vi "start.vi"(5 "FPS":dbl=1000.0, 6 "error in (no error)":errorcluster, 7 "Exposure (ms)":dbl=0.001, 8 "Cam id":u32, 9 "session in":refnum<k35>) -> (0 "error out":errorcluster, 1 "return value":T1={"x"=2592, "y"=1944, "FPS"=30.757874015748033, "Exposure"=0.027793333333333333}, 3 "session out":refnum<k35>)   [LabVIEW 2022 SP3]
panel:
  in  "Image Size template":T1={"x"=2592, "y"=1944, "FPS"=0.0, "Exposure"=0.0}
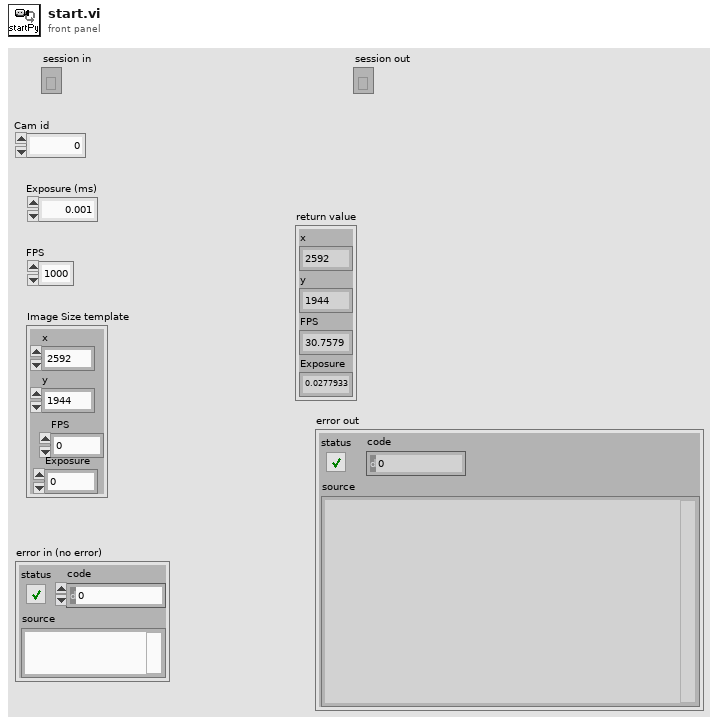
[diagram p1: front panel]
types:
  T1 = cluster{"x":i32, "y":i32, "FPS":dbl, "Exposure":dbl}
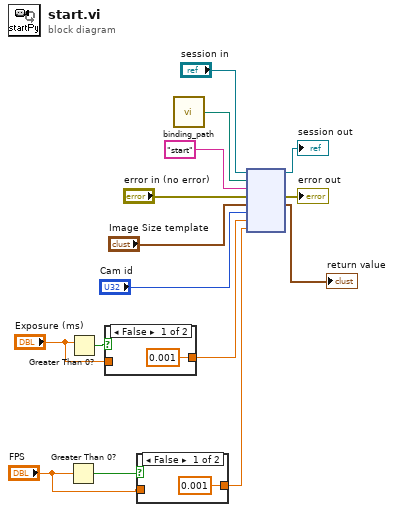
[diagram p0: block diagram]
diagram:
  n1 = Greater Than 0?(x="FPS") -> (x > 0?=w3:bool)
  n2 = Greater Than 0?(x="Exposure (ms)") -> (x > 0?=w6:bool)
  n3 = case shown="False" w6 {
    tunnel: [0.001 ("Exposure (ms)") w17] -> w5
    tunnel: "Exposure (ms)" -> [_ w17]
    frame False {
    }
    frame True {
    }
  }
  n4 = case shown="False" w3 {
    tunnel: [0.001 ("Exposure (ms)") w19] -> w1
    tunnel: "FPS" -> [_ w19]
    frame False {
    }
    frame True {
    }
  }
  n5 = call "binding_path.vi"() -> ("appended path"=w8:path)
  n6 = node("session in", w8, "start" ("function name"), "error in (no error)", "Image Size template", "Cam id", w5, w1) -> (→"session out":refnum<k35>, →"error out":errorcluster, →"return value":T1)  [unwired: 3 in, 2 out]
